vi "DimIndicators.application example any type.vi"() -> ()   [LabVIEW 2013, in "DimIndicators.lvlib"]
doc: "This VI demonstrates one possibility to subscribe to a DIM service via the DimIndicator library. You have to start the \"dim_operate\" VI of the LVDimInterface library as well as the \"dispatcher\" VI of this library before using this VI."
uses:
  DimIndicators.lvlib
  DimIndicators.anyType.ctl
panel:
  out "error out":errorcluster
  out "serviceData":string
  in  "serviceName":string="testService"
  in  "data":T1
  in  "stop":bool
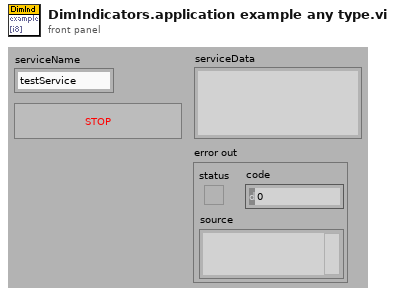
[diagram p1: front panel]
types:
  T1 = typedef "DimIndicators.lvlib/DimIndicators.anyType.ctl" = cluster{"data":string, "no link":bool, "quality":i32, "timeStamp":dbl}
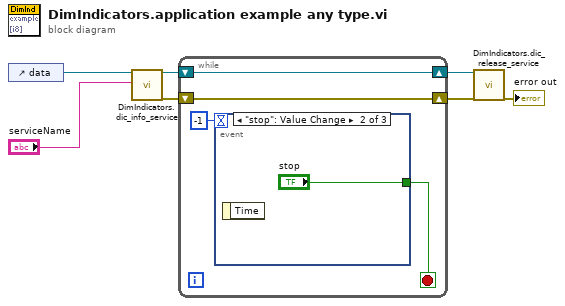
[diagram p0: block diagram]
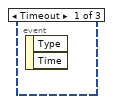
[diagram p2: hidden frame]
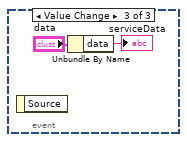
[diagram p3: hidden frame]
diagram:
  n1 = control-ref of="data"() -> (w4:refnum<vi>)
  n2 = call "DimIndicators.dic_info_service.vi"("controlRef"=w4, "serviceName"="serviceName") -> ("controlRef out"=w6:refnum<vi>, "error out"=w3:errorcluster)  [unwired: 16 in]
  n3 = while {
    shift-right: [w11] -> w5
    shift-left: w6 -> [w11]
    shift-right: [w8] -> w2
    shift-left: w3 -> [w8]
    stop <- w9 stop-if-true
    n4 = event shown="[1] \"stop\": Value Change" {
      selector: _ -> [_ _ _]
      dyn-events: _ -> [_ _ _]
      timeout: -1 -> [_ _ _]
      tunnel: [_ "stop" _] -> w9
      event Timeout {
        n5 = event-data() -> ()  [unwired: 1 in, 2 out]
      }
      event "stop": Value Change {
        n6 = event-data() -> ()  [unwired: 1 in, 1 out]
      }
      event Value Change {
        n7 = event-data() -> ()  [unwired: 1 in, 1 out]
        n8 = Unbundle By Name("data") -> ("data"=→"serviceData":string)
      }
    }
  }
  n9 = call "DimIndicators.dic_release_service.vi"("controlRef"=w5, "error in (no error)"=w2) -> ("error out"=→"error out":errorcluster)  [unwired: 17 in]
